vi "GetRobotModeFromControlWord.vi"(11 "Control Word":T1) -> (3 "Robot Mode":T2)   [LabVIEW 2020]
uses:
  <vilib>/Rock Robotics/WPI/DriverStation/WPI_DriverStationRobotMode2.ctl
  <vilib>/Rock Robotics/SystemInterfaces/NetworkCommunication/NetComm_ControlWord.ctl
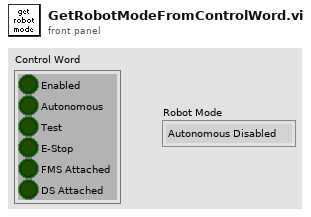
[diagram p1: front panel]
types:
  T1 = typedef "NetComm_ControlWord.ctl" = cluster{"Enabled":bool, "Autonomous":bool, "Test":bool, "E-Stop":bool, "FMS Attached":bool, "DS Attached":bool}
  T2 = typedef "WPI_DriverStationRobotMode2.ctl" = enum16{"Autonomous Disabled", "Autonomous Enabled", "Teleop Disabled", "Teleop Enabled", "Disconnected", "Finish", "Test Disabled", "Test Enabled", "Emergency Stopped"}
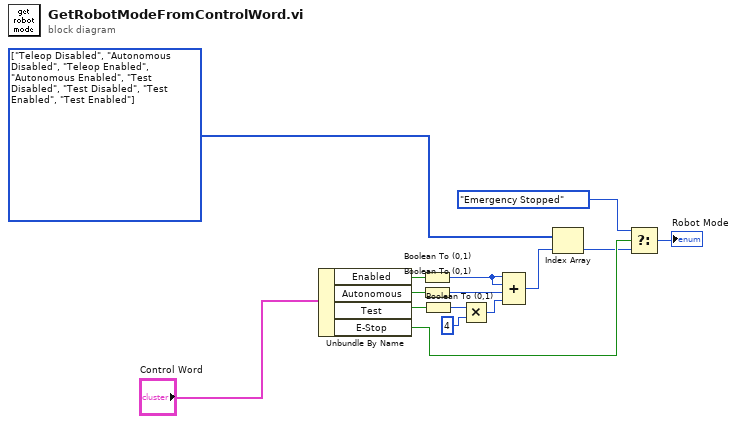
[diagram p0: block diagram]
diagram:
  w6 = T2[] [enum."Teleop Disabled", enum."Autonomous Disabled", enum."Teleop Enabled", enum."Autonomous Enabled", enum."Test Disabled", enum."Test Disabled", enum."Test Enabled", enum."Test Enabled"] items=["Autonomous Disabled", "Autonomous Enabled", "Teleop Disabled", "Teleop Enabled", "Disconnected", "Finish", "Test Disabled", "Test Enabled", "Emergency Stopped"]
  n1 = Unbundle By Name("Control Word") -> ("Enabled"=w13:bool, "Autonomous"=w14:bool, "Test"=w15:bool, "E-Stop"=w3:bool)
  n2 = Boolean To (0,1)(Boolean=w13) -> (0, 1=w8:i16)
  n3 = Boolean To (0,1)(Boolean=w14) -> (0, 1=w9:i16)
  n4 = Boolean To (0,1)(Boolean=w15) -> (0, 1=w11:i16)
  n5 = Multiply(x=w11, y=4) -> (x*y=w12:i32)
  n6 = Compound Arithmetic op=ADD(w8, w8, w9, w12) -> (w5:i32)
  n7 = Index Array(array=w6, index=w5) -> (element=w1:T2)
  n8 = Select(t=WPI_DriverStationRobotMode2."Emergency Stopped" ("RobotMode"), s=w3, f=w1) -> (s? t:f=→"Robot Mode":T2)
